vi "StdsXYGraph.vi"() -> (0 "Std Array":dbl[][](array[numeric]), 1 "Table":string[][](table), 2 "XY Graph":cluster{i32[], dbl[]}(graph), 3 "Stds Chart":dbl(graph))   [LabVIEW 2023]
panel:
  out "All Results":dbl[][](array[numeric])
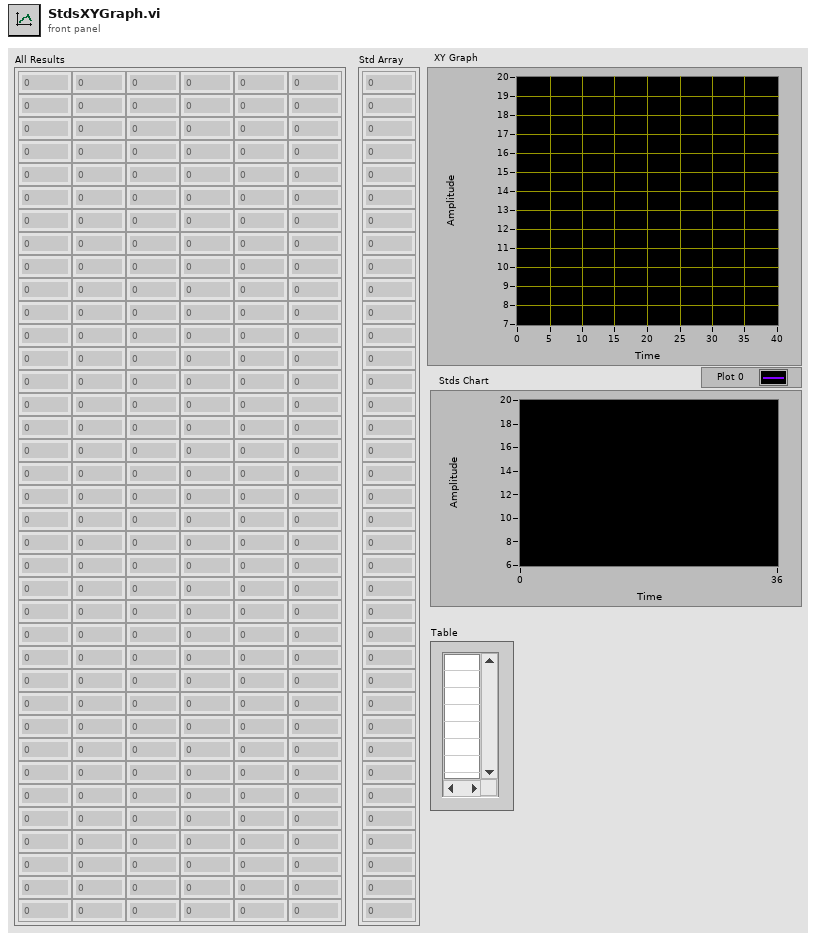
[diagram p1: front panel]
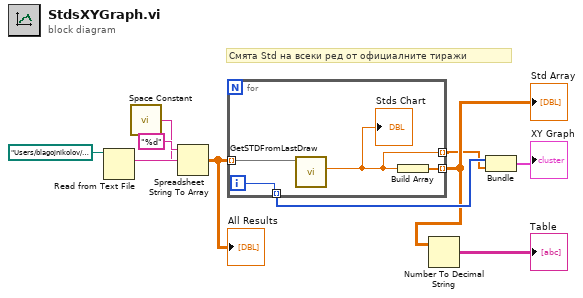
[diagram p0: block diagram]
diagram:
  # "Смята Std на всеки ред от официалните тиражи"
  n1 = Read from Text File(file (use dialog)=path "/Users/blagojnikolov/Desktop/@tmp/results.txt") -> (text=w9:string)  [unwired: 3 in, 3 out]
  n2 = call <vilib>:"Space Constant.vi"() -> ("String"=w7:string)
  n3 = Spreadsheet String To Array(delimiter (Tab)=w7, format string="%d", spreadsheet string=w9) -> (array=w6:dbl[][])  [unwired: 1 in]
  "All Results" <- w6
  n4 = for {
    tunnel: w6 -> [w13] mode=indexing
    tunnel: [w14] -> w3 mode=indexing
    tunnel: [w12] -> w4 mode=indexing
    tunnel: [w11] -> w1 mode=indexing
    i -> [w12]
    n5 = call "GetSTDFromLastDraw.vi"("Officials Results"=w13) -> ("STD"=w11:dbl)  [unwired: 8 in, 2 out]
    "Stds Chart" <- w11
    n6 = Build Array(w11) -> (w14:dbl[])
  }
  "Std Array" <- w3
  n7 = Number To Decimal String(number=w3) -> (decimal integer string=→"Table":string[][])  [unwired: 1 in]
  n8 = Bundle(w4, w1) -> (→"XY Graph":cluster{i32[], dbl[]})  [unwired: 1 in]
